vi "build_filename.vi"(9 "Test type":string, 10 "time stamp":timestamp, 11 "File config":cluster{"Filepath":path, "Test ID":string}) -> (3 "appended path":path)   [LabVIEW 2020]
panel:
  # "Build filename"
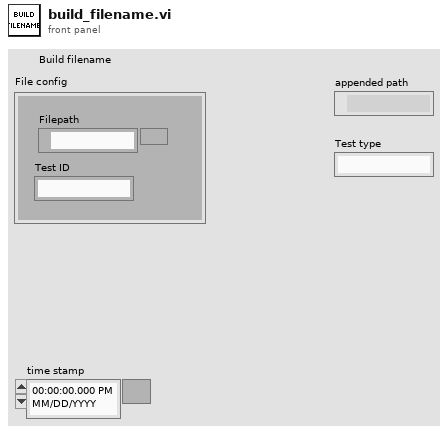
[diagram p1: front panel]
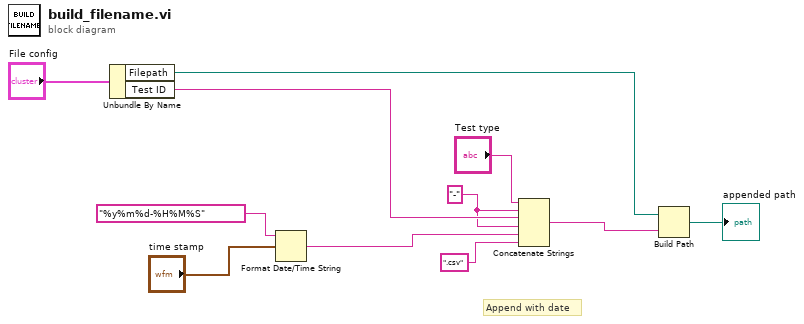
[diagram p0: block diagram]
diagram:
  w3 = "-" ("string")
  # "Append with date"
  n1 = Unbundle By Name("File config") -> ("Filepath"=w6:path, "Test ID"=w5:string)
  n2 = Format Date/Time String(time format string (%c)="%y%m%d-%H%M%S", seconds (now)="time stamp") -> (date/time string=w2:string)  [unwired: 1 in]
  n3 = Concatenate Strings("Test type", w3, w5, w3, w2, ".csv" ("Type")) -> (w11:string)
  n4 = Build Path(base path=w6, name or relative path=w11) -> (appended path=→"appended path":path)
